vi "vi to string file.vi"(4 "Export Diagram":bool, 6 "Create Captions":bool=TRUE, 8 "error in (no error)":errorcluster, 10 "String File Path in":path, 11 "VI Path in":path) -> (0 "error out":errorcluster, 2 "String File Path out":path, 3 "VI Path out":path)   [LabVIEW 2022 SP3]
doc: "This VI convert a .vi .ctl file into xml-like string file. The string file if exist will be replaced with new content."
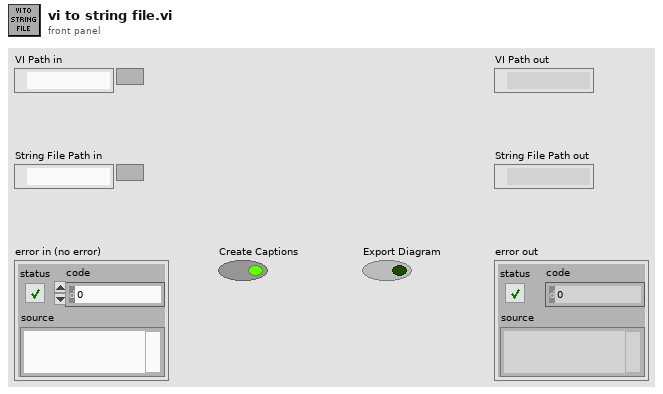
[diagram p1: front panel]
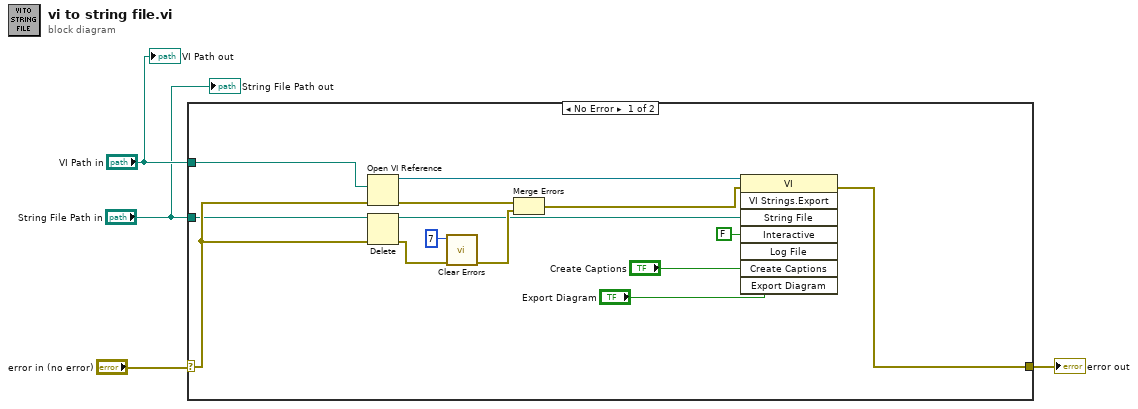
[diagram p0: block diagram]
diagram:
  n1 = case shown="No Error" "error in (no error)" {
    selector: "error in (no error)" -> [w11 w19]
    tunnel: [w14 w19] -> w4
    tunnel: "VI Path in" -> [w7 _]
    tunnel: "String File Path in" -> [w6 _]
    frame No Error {
      n2 = Open VI Reference(vi path=w7, error in (no error)=w11) -> (vi reference=w18:refnum<vi>, error out=w10:errorcluster)  [unwired: 4 in]
      n3 = Delete(path (use dialog)=w6, error in=w11) -> (deleted path=w5:path, error out=w12:errorcluster)  [unwired: 3 in, 1 out]
      n4 = call <vilib>:"Clear Errors.vi"("error in (no error)"=w12, "specific error code to clear (0: all)"=7) -> ("error out"=w9:errorcluster)  [unwired: 4 in, 1 out]
      n5 = Merge Errors(w10, w9) -> (w8:errorcluster)
      n6 = invoke class="VI" method="VI Strings.Export"(reference=w18, error in=w8, "String File"=w5, "Interactive"=FALSE, "Create Captions"="Create Captions", "Export Diagram"="Export Diagram") -> (error out=w14:errorcluster)  [unwired: 2 in, 7 out]
    }
    frame Error {
    }
  }
  "error out" <- w4
  "VI Path out" <- "VI Path in"
  "String File Path out" <- "String File Path in"
